vi "LS340_ConfigCtrlParam.vi"(0 "VISA resource name":refnum<visa-resource-name>, 1 "Manual Output (0.00)":dbl min=0.0 max=100.0 step=0.01 format="%.2f", 2 "Heater Range (0: Off)":u16(ring) items=["Off", "1", "2", "3", "4", "5"], 5 "Loop (0: 1)":u16(ring) items=["1", "2"], 7 "Gain (P) (0.0)":dbl min=0.0 max=1000.0 step=0.1 format="%.1f", 9 "Reset (I) (0.0)":dbl min=0.0 max=1000.0 step=0.1 format="%.1f", 11 "error in (no error)":errorcluster, 12 "Rate (D) (0)":dbl min=0.0 max=1000.0 step=1.0) -> (4 "VISA resource name out":refnum<visa-resource-name>, 15 "error out":errorcluster)   [LabVIEW 2012]
doc: "This VI Configures the 340 Control Parameters, functions configured are PID, Heater Range, and Manual Output."
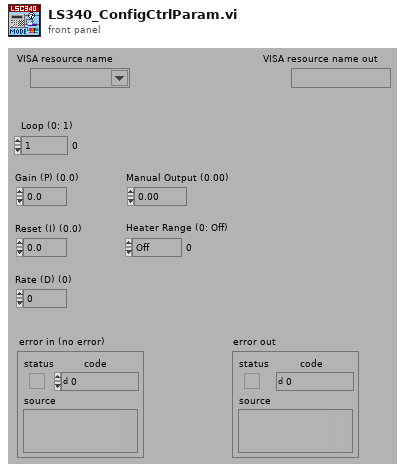
[diagram p1: front panel]
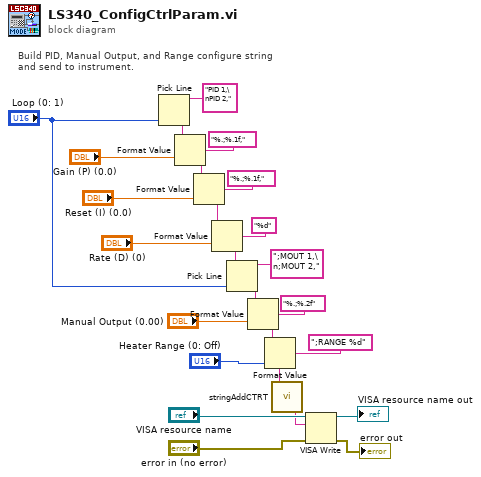
[diagram p0: block diagram]
diagram:
  # "Build PID, Manual Output, and Range configure string\nand send to instrument."
  n1 = Pick Line(multi-line string="PID 1,\nPID 2,", line index="Loop (0: 1)") -> (output string=w20:string)  [unwired: 1 in]
  n2 = Format Value(string ("")=w20, format string="%.;%.1f,", value (0)="Gain (P) (0.0)") -> (output string=w19:string)
  n3 = Format Value(string ("")=w19, format string="%.;%.1f,", value (0)="Reset (I) (0.0)") -> (output string=w18:string)
  n4 = Format Value(string ("")=w18, format string="%d", value (0)="Rate (D) (0)") -> (output string=w13:string)
  n5 = Pick Line(string ("")=w13, multi-line string=";MOUT 1,\n;MOUT 2,", line index="Loop (0: 1)") -> (output string=w9:string)
  n6 = Format Value(string ("")=w9, format string="%.;%.2f", value (0)="Manual Output (0.00)") -> (output string=w7:string)
  n7 = Format Value(string ("")=w7, format string=";RANGE %d", value (0)="Heater Range (0: Off)") -> (output string=w6:string)
  n8 = call "stringAddCTRT.vi"("string"=w6) -> ("strOut"=w1:string)  [unwired: 2 in]
  n9 = VISA Write(VISA resource name="VISA resource name", write buffer=w1, error in (no error)="error in (no error)") -> (VISA resource name out=→"VISA resource name out":refnum<visa-resource-name>, error out=→"error out":errorcluster)  [unwired: 1 out]
